vi "zlgcan_receive.vi"(2 "输入字符串":string, 3 "协议":u8, 4 "通道句柄":u32) -> (0 "输出字符串":string, 1 "结果":bool)   [LabVIEW 2017]
uses:
  bin/zlgcan_wrap.dll
panel:
  out "临时":string
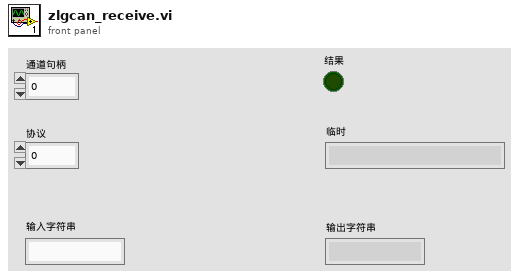
[diagram p1: front panel]
types:
  T1 = cluster{"[0]":u8, "[1]":u8, "[2]":u8, "[3]":u8, "[4]":u8, "[5]":u8, "[6]":u8, "[7]":u8}
  T2 = cluster{u32, u8, u8, u8, u8, cluster{"[0]":u8, "[1]":u8, "[2]":u8, "[3]":u8, "[4]":u8, "[5]":u8, "[6]":u8, "[7]":u8}, u64}
  T3 = cluster{u32, u8, u8, u8, u8, cluster{"[0]":u8, "[1]":u8, "[2]":u8, "[3]":u8, "[4]":u8, "[5]":u8, "[6]":u8, "[7]":u8}, u64}[]
  T4 = cluster{"[0]":u8, "[1]":u8, "[2]":u8, "[3]":u8, "[4]":u8, "[5]":u8, "[6]":u8, "[7]":u8, "[8]":u8, "[9]":u8, "[10]":u8, "[11]":u8, "[12]":u8, "[13]":u8, "[14]":u8, "[15]":u8, "[16]":u8, "[17]":u8, "[18]":u8, "[19]":u8, "[20]":u8, "[21]":u8, "[22]":u8, "[23]":u8, "[24]":u8, "[25]":u8, "[26]":u8, "[27]":u8, "[28]":u8, "[29]":u8, "[30]":u8, "[31]":u8, "[32]":u8, "[33]":u8, "[34]":u8, "[35]":u8, "[36]":u8, "[37]":u8, "[38]":u8, "[39]":u8, "[40]":u8, "[41]":u8, "[42]":u8, "[43]":u8, "[44]":u8, "[45]":u8, "[46]":u8, "[47]":u8, "[48]":u8, "[49]":u8, "[50]":u8, "[51]":u8, "[52]":u8, "[53]":u8, "[54]":u8, "[55]":u8, "[56]":u8, "[57]":u8, "[58]":u8, "[59]":u8, "[60]":u8, "[61]":u8, "[62]":u8, "[63]":u8}
  T5 = cluster{u32, u8, u8, u8, u8, cluster{"[0]":u8, "[1]":u8, "[2]":u8, "[3]":u8, "[4]":u8, "[5]":u8, "[6]":u8, "[7]":u8, "[8]":u8, "[9]":u8, "[10]":u8, "[11]":u8, "[12]":u8, "[13]":u8, "[14]":u8, "[15]":u8, "[16]":u8, "[17]":u8, "[18]":u8, "[19]":u8, "[20]":u8, "[21]":u8, "[22]":u8, "[23]":u8, "[24]":u8, "[25]":u8, "[26]":u8, "[27]":u8, "[28]":u8, "[29]":u8, "[30]":u8, "[31]":u8, "[32]":u8, "[33]":u8, "[34]":u8, "[35]":u8, "[36]":u8, "[37]":u8, "[38]":u8, "[39]":u8, "[40]":u8, "[41]":u8, "[42]":u8, "[43]":u8, "[44]":u8, "[45]":u8, "[46]":u8, "[47]":u8, "[48]":u8, "[49]":u8, "[50]":u8, "[51]":u8, "[52]":u8, "[53]":u8, "[54]":u8, "[55]":u8, "[56]":u8, "[57]":u8, "[58]":u8, "[59]":u8, "[60]":u8, "[61]":u8, "[62]":u8, "[63]":u8}, u64}
  T6 = cluster{u32, u8, u8, u8, u8, cluster{"[0]":u8, "[1]":u8, "[2]":u8, "[3]":u8, "[4]":u8, "[5]":u8, "[6]":u8, "[7]":u8, "[8]":u8, "[9]":u8, "[10]":u8, "[11]":u8, "[12]":u8, "[13]":u8, "[14]":u8, "[15]":u8, "[16]":u8, "[17]":u8, "[18]":u8, "[19]":u8, "[20]":u8, "[21]":u8, "[22]":u8, "[23]":u8, "[24]":u8, "[25]":u8, "[26]":u8, "[27]":u8, "[28]":u8, "[29]":u8, "[30]":u8, "[31]":u8, "[32]":u8, "[33]":u8, "[34]":u8, "[35]":u8, "[36]":u8, "[37]":u8, "[38]":u8, "[39]":u8, "[40]":u8, "[41]":u8, "[42]":u8, "[43]":u8, "[44]":u8, "[45]":u8, "[46]":u8, "[47]":u8, "[48]":u8, "[49]":u8, "[50]":u8, "[51]":u8, "[52]":u8, "[53]":u8, "[54]":u8, "[55]":u8, "[56]":u8, "[57]":u8, "[58]":u8, "[59]":u8, "[60]":u8, "[61]":u8, "[62]":u8, "[63]":u8}, u64}[]
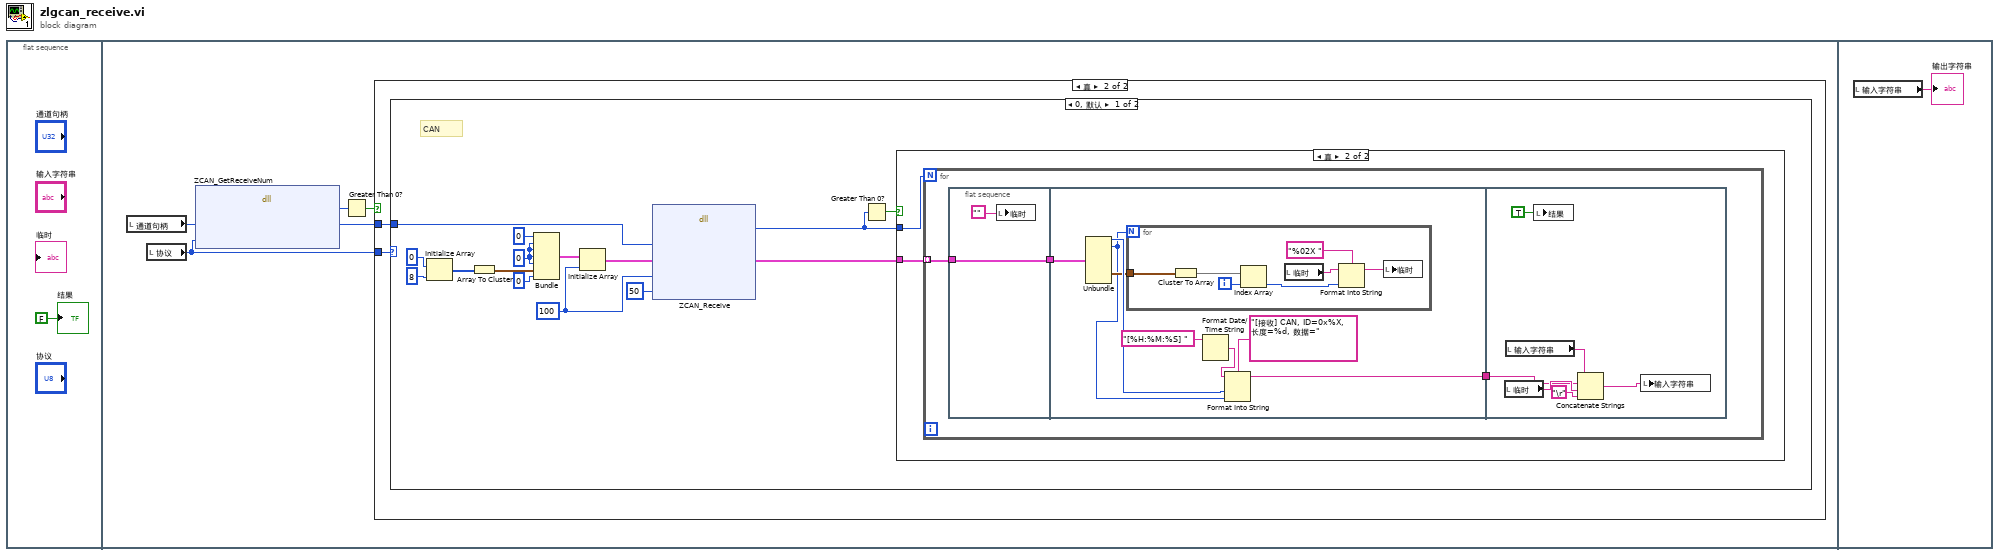
[diagram p0: block diagram]
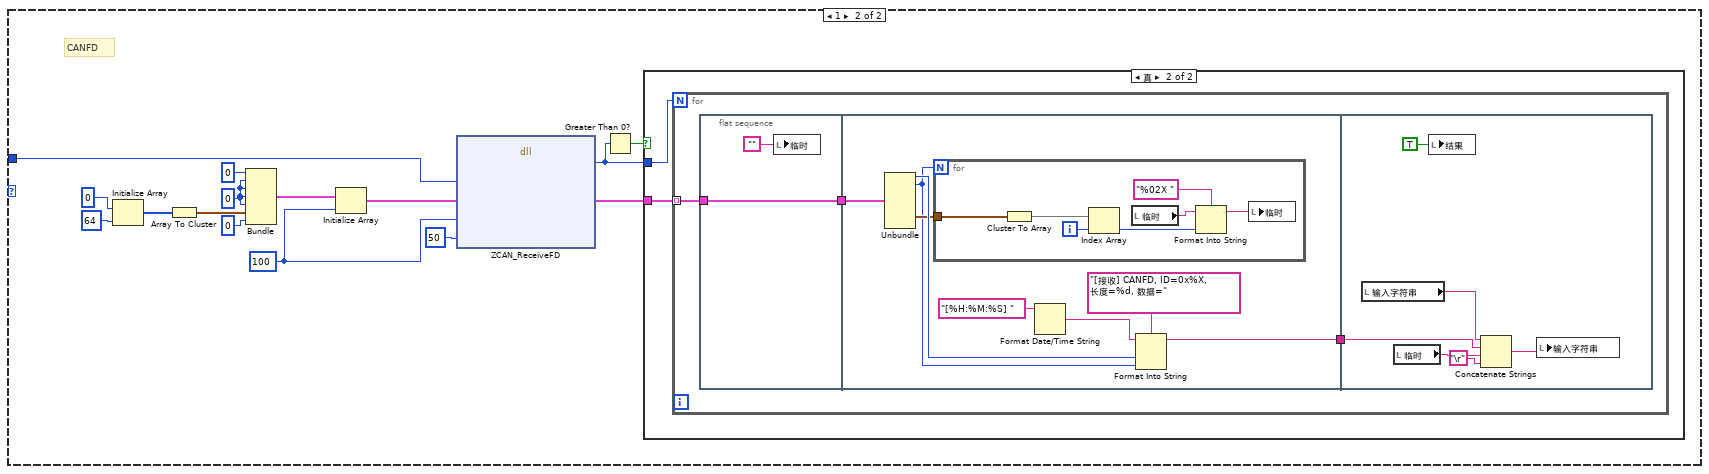
[diagram p4: hidden frame]
diagram:
  n1 = flat-sequence {
    frame #0 {
      "结果" <- FALSE ("结果")
    }
    frame #1 {
      n2 = local read "通道句柄"() -> (w4:u32)
      n3 = local read "协议"() -> (w2:u8)
      n4 = dll-call lib="E:/Project/CANMaster/LabView/ZlgCan_Demo/bin/zlgcan_wrap.dll" fn="ZCAN_GetReceiveNum"("通道句柄"=w4, "协议"=w2) -> ("返回类型"=w6:u32, "通道句柄"=w3:u32)  [unwired: 4 in, 2 out]
      n5 = Greater Than 0?(x=w6) -> (x > 0?=w5:bool)
      n6 = case shown="真" w5 {
        tunnel: w3 -> [_ w8]
        tunnel: w2 -> [_ w7]
        frame False {
        }
        frame True {
          n7 = case shown="0, 默认" w7 {
            tunnel: w8 -> [w23 w66]
            frame 0, Default {
              w18 = u8 0
              w13 = 100 ("维数大小")
              # "CAN"
              n8 = Initialize Array(u8 0 ("元素"), u32 8 ("维数大小")) -> (w20:u8[])
              n9 = Array To Cluster(array=w20) -> (cluster=w21:T1)
              n10 = Bundle(u32 0, w18, w18, w18, w18, w21, u64 0) -> (w22:T2)  [unwired: 1 in]
              n11 = Initialize Array(w22, w13) -> (w12:T3)
              n12 = dll-call lib="E:/Project/CANMaster/LabView/ZlgCan_Demo/bin/zlgcan_wrap.dll" fn="ZCAN_Receive"("通道句柄"=w23, "数据帧数组"=w12, "数据帧数"=w13, "超时时间"=50) -> ("返回类型"=w10:u32, "数据帧数组"=w9:T3)  [unwired: 6 in, 2 out]
              n13 = Greater Than 0?(x=w10) -> (x > 0?=w11:bool)
              n14 = case shown="真" w11 {
                tunnel: w10 -> [_ w24]
                tunnel: w9 -> [_ w25]
                frame False {
                }
                frame True {
                  n15 = for {
                    N: w24 -> [_]
                    tunnel: w25 -> [w28] mode=indexing
                    n16 = flat-sequence {
                      tunnel: w28 -> [w30]
                      tunnel: [w30] -> w26
                      tunnel: [w37] -> w27
                      tunnel: w26 -> [w38]
                      tunnel: w27 -> [w47]
                      frame #0 {
                        n17 = local write "临时"("") -> ()
                      }
                      frame #1 {
                        n18 = Unbundle(w38) -> (w36:u32, w34:u8, w35:T1)  [unwired: 4 out]
                        n19 = for {
                          N: w34 -> [_]
                          tunnel: w35 -> [w45]
                          i -> [w43]
                          n20 = Cluster To Array(cluster=w45) -> (array=w44:u8[])
                          n21 = Index Array(array=w44, index=w43) -> (element=w41:u8)
                          n22 = local read "临时"() -> (w40:string)
                          n23 = Format Into String(format string="%02X " ("格式字符串"), initial string=w40, w41) -> (resulting string=w39:string)  [unwired: 1 in, 1 out]
                          n24 = local write "临时"(w39) -> ()
                        }
                        n25 = Format Date/Time String(time format string (%c)="[%H:%M:%S] " ("时间格式字符串(%c)")) -> (date/time string=w31:string)  [unwired: 2 in]
                        n26 = Format Into String(format string="[接收] CAN, ID=0x%X, 长度=%d, 数据=" ("格式字符串"), initial string=w31, w36, w34) -> (resulting string=w37:string)  [unwired: 1 in, 1 out]
                      }
                      frame #2 {
                        n27 = local read "临时"() -> (w50:string)
                        n28 = local read "输入字符串"() -> (w46:string)
                        n29 = local write "结果"(TRUE ("结果")) -> ()
                        n30 = Concatenate Strings(w46, w47, w50, "\r") -> (w48:string)
                        n31 = local write "输入字符串"(w48) -> ()
                      }
                    }
                  }
                }
              }
            }
            frame 1 {
              w61 = u8 0
              w55 = 100 ("维数大小")
              # "CANFD"
              n32 = Initialize Array(u8 0 ("元素"), u32 64 ("维数大小")) -> (w63:u8[])
              n33 = Array To Cluster(array=w63) -> (cluster=w64:T4)
              n34 = Bundle(u32 0, w61, w61, w61, w61, w64, u64 0) -> (w65:T5)  [unwired: 1 in]
              n35 = Initialize Array(w65, w55) -> (w57:T6)
              n36 = dll-call lib="E:/Project/CANMaster/LabView/ZlgCan_Demo/bin/zlgcan_wrap.dll" fn="ZCAN_ReceiveFD"("通道句柄"=w66, "数据帧数组"=w57, "数据帧数"=w55, "超时时间"=50) -> ("返回类型"=w53:u32, "数据帧数组"=w54:T6)  [unwired: 6 in, 2 out]
              n37 = Greater Than 0?(x=w53) -> (x > 0?=w52:bool)
              n38 = case shown="真" w52 {
                tunnel: w54 -> [_ w68]
                tunnel: w53 -> [_ w67]
                frame False {
                }
                frame True {
                  n39 = for {
                    N: w67 -> [_]
                    tunnel: w68 -> [w71] mode=indexing
                    n40 = flat-sequence {
                      tunnel: w71 -> [w73]
                      tunnel: [w73] -> w69
                      tunnel: [w80] -> w70
                      tunnel: w69 -> [w81]
                      tunnel: w70 -> [w90]
                      frame #0 {
                        n41 = local write "临时"("") -> ()
                      }
                      frame #1 {
                        n42 = Unbundle(w81) -> (w79:u32, w77:u8, w78:T4)  [unwired: 4 out]
                        n43 = for {
                          N: w77 -> [_]
                          tunnel: w78 -> [w88]
                          i -> [w86]
                          n44 = Cluster To Array(cluster=w88) -> (array=w87:u8[])
                          n45 = Index Array(array=w87, index=w86) -> (element=w84:u8)
                          n46 = local read "临时"() -> (w83:string)
                          n47 = Format Into String(format string="%02X " ("格式字符串"), initial string=w83, w84) -> (resulting string=w82:string)  [unwired: 1 in, 1 out]
                          n48 = local write "临时"(w82) -> ()
                        }
                        n49 = Format Date/Time String(time format string (%c)="[%H:%M:%S] " ("时间格式字符串(%c)")) -> (date/time string=w74:string)  [unwired: 2 in]
                        n50 = Format Into String(format string="[接收] CANFD, ID=0x%X, 长度=%d, 数据=" ("格式字符串"), initial string=w74, w79, w77) -> (resulting string=w80:string)  [unwired: 1 in, 1 out]
                      }
                      frame #2 {
                        n51 = local read "输入字符串"() -> (w89:string)
                        n52 = local read "临时"() -> (w93:string)
                        n53 = local write "结果"(TRUE ("结果")) -> ()
                        n54 = Concatenate Strings(w89, w90, w93, "\r") -> (w91:string)
                        n55 = local write "输入字符串"(w91) -> ()
                      }
                    }
                  }
                }
              }
            }
          }
        }
      }
    }
    frame #2 {
      n56 = local read "输入字符串"() -> (→"输出字符串":string)
    }
  }
